vi "luaL_newstate.vi"(8 "error in (no error)":errorcluster) -> (0 "error out":errorcluster, 3 "lua_state_p":u64)   [LabVIEW 2020, in "lua.dll.lvlib"]
doc: "luaL_newstate\n[-0, +0, –]\nlua_State *luaL_newstate (void);\nCreates a new Lua state. It calls lua_newstate with an allocator based on the standard C allocation functions and then sets a warning function and a panic function (see §4.4) that print messages to the standard error output.\n\nReturns the new state, or NULL if there is a memory allocation error."
uses:
  lua.dll.lvlib
  lua54.dll
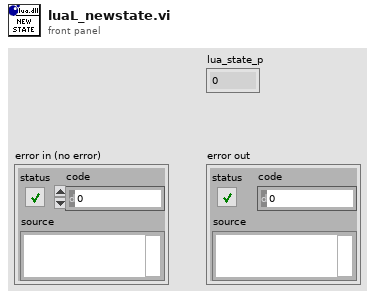
[diagram p1: front panel]
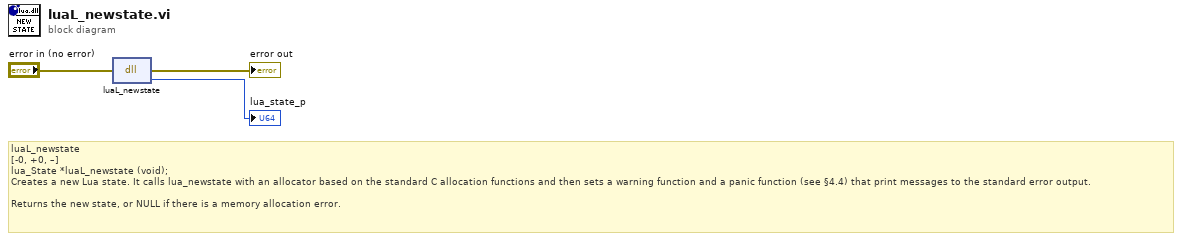
[diagram p0: block diagram]
diagram:
  # "luaL_newstate\n[-0, +0, –]\nlua_State *luaL_newstate (void);\nCreates a new Lua state. It calls lua_newstate with an allocator based on the standard C allocation functions and then sets a warning function and a panic function (see §4.4) that print messages to the standard error output.\n\nReturns the new state, or NULL if there is a memory allocation error."
  n1 = dll-call lib="C:/Users/Nicholas Folse/Documents/workspace/github-tauterra.llc/Lua for LabVIEW/lib/lua.dll/lua54**.*" fn="luaL_newstate"(error in="error in (no error)") -> (error out=→"error out":errorcluster, "lua_state_p"=→"lua_state_p":u64)  [unwired: 2 in, 1 out]
